vi "Format MCLI Configuration Log.vi"(8 "error in (no error)":errorcluster, 11 "Instrument.Lockin in":refnum<class "Instrument.Lockin.lvclass">) -> (0 "error out":errorcluster, 1 "Log Data":T1[](array[typedef]), 2 "Log Paths":string, 3 "Instrument.Lockin out":refnum<class "Instrument.Lockin.lvclass">, 4 "Times":timestamp[](array[timestamp]))   [LabVIEW 2019, in "Instrument.Lockin.lvlib" / "Instrument.Lockin.lvclass"]
uses:
  Instrument.Lockin.lvclass
  Typedefs/Lockin.LogConfiguration.MCLI--Cluster.ctl
  Instrument.Lockin.lvclass/Instrument.Lockin.ctl
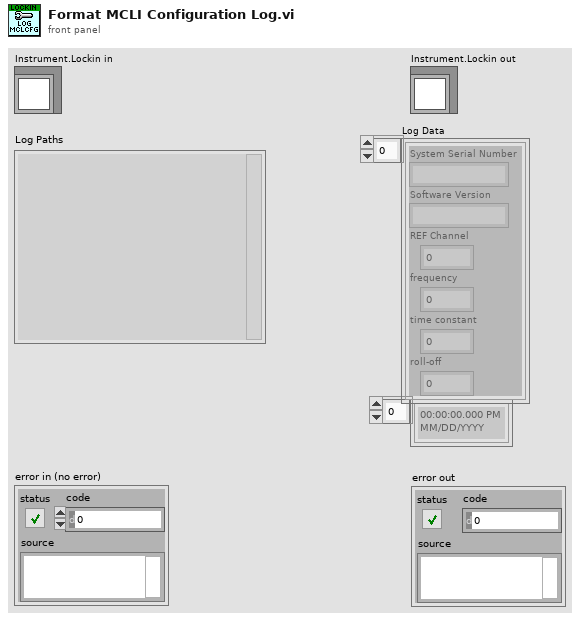
[diagram p1: front panel]
types:
  T1 = typedef "Instrument.Lockin.lvlib/Instrument.Lockin.lvclass/Lockin.LogConfiguration.MCLI--Cluster.ctl" = cluster{"System Serial Number":string, "Software Version":string, "REF Channel":i32, "frequency":dbl, "time constant":dbl, "roll-off":i32}
  T2 = typedef "Instrument.Lockin.lvlib/Instrument.DAQ.lvclass/REF.Channel--Cluster--Array.ctl" = T3[]
  T3 = typedef "Instrument.Lockin.lvlib/Instrument.DAQ.lvclass/REF.Channel--Cluster.ctl" = cluster{"Enable?":bool, "Channel":i32, "Frequency":dbl, "Phase":dbl, "TC":dbl, "Roll-Off":i32}
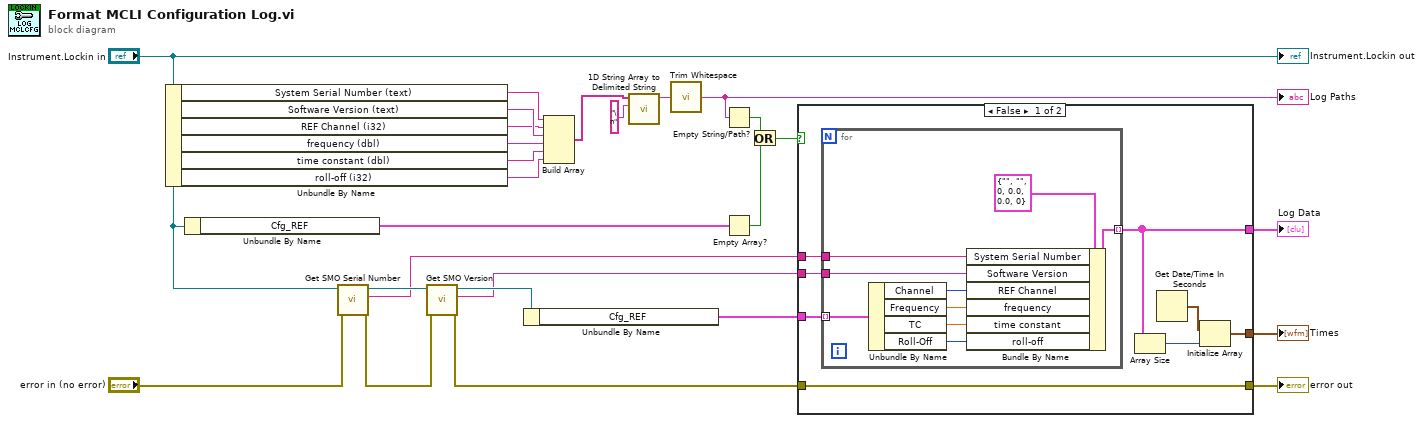
[diagram p0: block diagram]
diagram:
  n1 = Unbundle By Name("Instrument.Lockin in") -> ("System Serial Number (text)"=w25:string, "Software Version (text)"=w6:string, "REF Channel (i32)"=w5:string, "frequency (dbl)"=w4:string, "time constant (dbl)"=w3:string, "roll-off (i32)"=w2:string)
  n2 = Unbundle By Name("Instrument.Lockin in") -> ("Cfg_REF"=w15:T2)
  n3 = call-dynamic "Get SMO Serial Number.vi"("error in (no error)"="error in (no error)", "Instrument.Lockin in"="Instrument.Lockin in") -> ("error out"=w13:errorcluster, "Serial Number"=w11:string, "Instrument.Lockin out"=w14:refnum<class "Instrument.Lockin.lvclass">)  [unwired: 7 in]
  n4 = call-dynamic "Get SMO Version.vi"("error in (no error)"=w13, "Instrument.Lockin in"=w14) -> ("error out"=w12:errorcluster, "Version"=w9:string, "Instrument.Lockin out"=w10:refnum<class "Instrument.Lockin.lvclass">)  [unwired: 7 in]
  n5 = Unbundle By Name(w10) -> ("Cfg_REF"=w8:T2)
  n6 = Build Array(w25, w5, w6, w4, w3, w2) -> (w24:string[])
  n7 = call <vilib>:"1D String Array to Delimited String.vi"("delimiter"="\n", "string array"=w24) -> ("delimited string"=w18:string)  [unwired: 9 in]
  n8 = call <vilib>:"Trim Whitespace.vi"("string"=w18) -> ("trimmed string"=w17:string)  [unwired: 1 in]
  "Log Paths" <- w17
  n9 = Empty String/Path?(string/path=w17) -> (empty?=w20:bool)
  n10 = Empty Array?(array=w15) -> (empty?=w21:bool)
  n11 = Or(x=w20, y=w21) -> (x .or. y?=w19:bool)
  n12 = case shown="False" w19 {
    tunnel: [w27 _] -> w26
    tunnel: [w31 _] -> w7
    tunnel: w12 -> [w28 w44]
    tunnel: w11 -> [w34 _]
    tunnel: [w28 w44] -> w22
    tunnel: w9 -> [w33 _]
    tunnel: w8 -> [w32 _]
    frame False {
      n13 = for {
        tunnel: [w41] -> w31 mode=indexing
        tunnel: w34 -> [w43]
        tunnel: w33 -> [w42]
        tunnel: w32 -> [w39] mode=indexing
        n14 = Unbundle By Name(w39) -> ("Channel"=w38:i32, "Frequency"=w35:dbl, "TC"=w36:dbl, "Roll-Off"=w37:i32)
        n15 = Bundle By Name(cluster=T1 {"System Serial Number"="", "Software Version"="", "REF Channel"=0, "frequency"=0.0, "time constant"=0.0, "roll-off"=0} ("MCLI Configuration"), "System Serial Number"=w43, "Software Version"=w42, "REF Channel"=w38, "frequency"=w35, "time constant"=w36, "roll-off"=w37) -> (w41:T1)
      }
      n16 = Array Size(array=w31) -> (size(s)=w30:i32)
      n17 = Get Date/Time In Seconds() -> (seconds since 1Jan1904=w29:timestamp)
      n18 = Initialize Array(w29, w30) -> (w27:timestamp[])
    }
    frame True {
    }
  }
  "Times" <- w26
  "error out" <- w22
  "Log Data" <- w7
  "Instrument.Lockin out" <- "Instrument.Lockin in"
